vi "Sequence Start.vi"(8 "error in (no error)":errorcluster, 11 "MSX-E3711 in":refnum<class "MSX-E3711.lvclass">) -> (0 "error out":errorcluster, 3 "MSX-E3711 out":refnum<class "MSX-E3711.lvclass">)   [LabVIEW 2014, in "MSX-E3711.lvlib" / "MSX-E3711.lvclass"]
uses:
  MSX-E3711.lvclass
  MSX-E3711.lvclass/MSX-E3711.ctl
  DriverMasterSync/build/DriverMasterSync.lvlibp/Modules/HAL/DriverMasterSync/DriverMasterSyncClass/DriverMasterSync.lvclass
  API/MSX-E3711_dll.lvlib
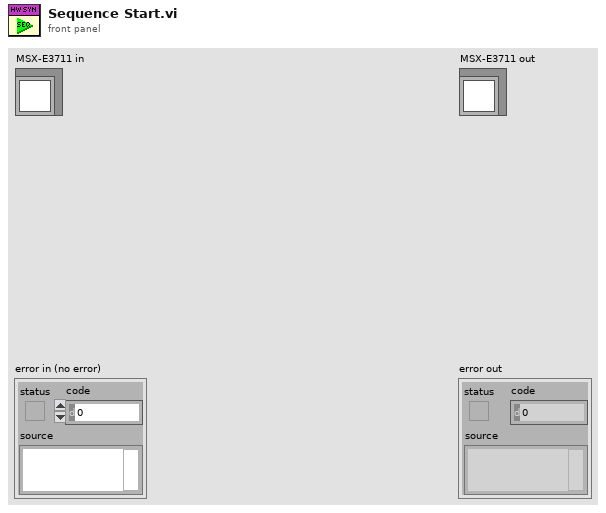
[diagram p1: front panel]
types:
  T1 = typedef "DriverMasterSync.lvlibp/HAL Config Data.ctl" = cluster{"HWSync Index":u32, "Driver Name":string, "Channel Mask":u64}
  T2 = typedef "MSX-E3711_dll.lvlib/Connection Data.ctl" = cluster{"MX371x refnum":refnum<k24>, "IP":string, "Connection ID ":refnum<k5>, "MXCommon refnum":refnum<k24>}
  T3 = typedef "MSX-E3711_dll.lvlib/Config Data.ctl" = cluster{"Auto Refresh":cluster{"Average Mode":u64, "Average Value":u64, "Trigger Mask":u64, "Trigger Mode":u64, "Hardware Trigger Edge":u64, "Hardware Trigger Count":u64, "By Trigger Nbr Of Seq To Acquire":u64, "Time stamp":bool, "Analog Output(mm)":bool, "Invert value":bool, "Temperature value":bool, "Incremental counter value":bool, "Diff. mode":bool}, "Gain":sgl[], "Offset":sgl[], "Index":u64, "Range":sgl, "Sequence":cluster{"Nbr Of Sequence":u64, "Nbr Max Sequence To Transfer":u64, "Delay Mode":u64, "Delay Time Unit":u64, "Delay Value":u64, "Trigger Mask":u64, "Trigger Mode":u64, "Hardware Trigger Edge":u64, "Hardware Trigger Count":u64, "By Trigger Nbr Of Seq To Acquire":u64, "Time stamp":bool, "Sequence counter information":bool, "Analog Output(mm)":bool, "Invert value":bool, "Temperature value":bool, "Incremental counter value":bool, "Diff. mode":bool}, "Enable DIO":bool, "IncCounter":cluster{"CounterMode":string, "CounterOptionDIRECT  ":bool, "CounterOptionOthers":bool, "CounterClear ":bool, "Cantidad de Pulsos":sgl, "Reducción":sgl}, "IncTemperature":cluster{"ConnectedTempSensor":string, "ConvertMode":string, "InitGainSelection":string, "FrequencySelection":string, "PowerSaveMode":bool, "GainSelection":string, "RefValue":dbl}}
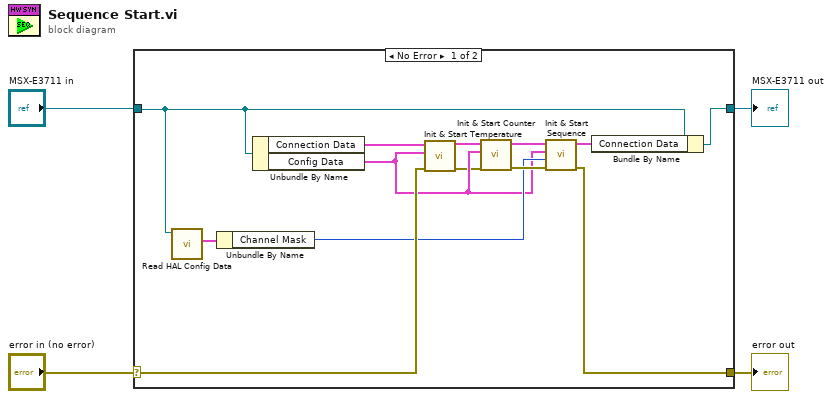
[diagram p0: block diagram]
diagram:
  n1 = case shown="No Error" "error in (no error)" {
    selector: "error in (no error)" -> [w13 w19]
    tunnel: [w11 w19] -> w3
    tunnel: [w15 w18] -> w1
    tunnel: "MSX-E3711 in" -> [w14 w18]
    frame No Error {
      n2 = call "Read HAL Config Data.vi"("DriverMasterSync in"=w14) -> ("HAL Config Data"=w17:T1)  [unwired: 8 in, 2 out]
      n3 = Unbundle By Name(w17) -> ("Channel Mask"=w9:u64)
      n4 = Unbundle By Name(w14) -> ("Connection Data"=w16:T2, "Config Data"=w8:T3)
      n5 = call "Init & Start Temperature.vi"("error in (no error)"=w13, "Config Data"=w8, "Connection Data In"=w16) -> ("error out"=w6:errorcluster, "Connection Data Out"=w5:T2)  [unwired: 7 in]
      n6 = call "Init & Start Counter.vi"("error in (no error)"=w6, "Config Data"=w8, "Connection Data In"=w5) -> ("error out"=w10:errorcluster, "Connection Data Out"=w7:T2)  [unwired: 7 in]
      n7 = call "Init & Start Sequence.vi"("error in (no error)"=w10, "Channel Mask"=w9, "Config Data"=w8, "Connection Data In"=w7) -> ("error out"=w11:errorcluster, "Connection Data Out"=w12:T2)  [unwired: 6 in]
      n8 = Bundle By Name(cluster=w14, "Connection Data"=w12) -> (w15:refnum<class "MSX-E3711.lvclass">)
    }
    frame Error {
    }
  }
  "error out" <- w3
  "MSX-E3711 out" <- w1
